vi "Method One Return Value.vi"(8 "error in (no error)":errorcluster, 11 "Test Interface Mock in":refnum<class "Test Interface Pure Mock.lvclass">) -> (0 "error out":errorcluster, 2 "Return Value":dbl, 3 "Test Interface Mock out":refnum<class "Test Interface Pure Mock.lvclass">)   [LabVIEW 2020, in "Test Interface Pure Mock.lvclass"]
uses:
  Test Interface Pure Mock.lvclass
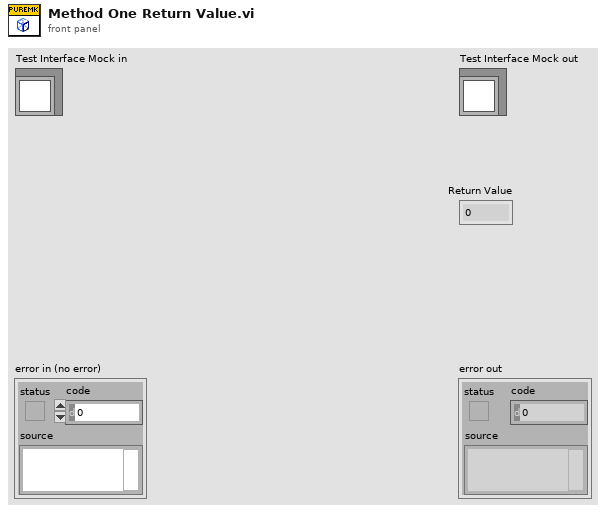
[diagram p1: front panel]
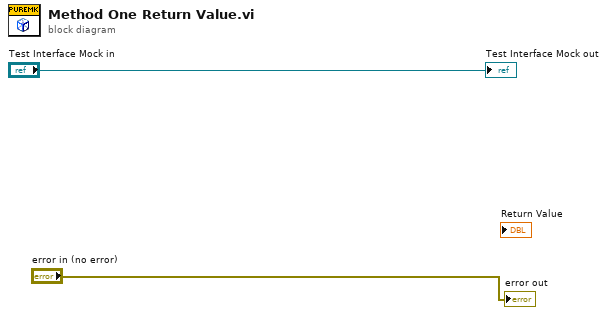
[diagram p0: block diagram]
diagram:
  "error out" <- "error in (no error)"
  "Test Interface Mock out" <- "Test Interface Mock in"
